vi "set dimmer.vi"(8 "error in":errorcluster, 10 "Set Dim":bool, 11 "Set Max Dim":bool) -> (0 "error out":errorcluster, 3 "Dim Level":T3 scale=0.0..100.0)   [LabVIEW 2013]
uses:
  Controls/Dim level.ctl
  Controls/Power Values.ctl
  <vilib>/addons/Electrical Power/Basic/Measurement/subVIs/basic_Power Value.ctl
  <vilib>/DAQmx/read.llb/DAQmx Read (Analog 1D Wfm NChan NSamp).vi
  <vilib>/addons/Electrical Power/Basic/Measurement/Power (1 Channel).vi
  <vilib>/DAQmx/miscellaneous.llb/DAQmx Fill In Error Info.vi
  <vilib>/addons/Electrical Power/Basic/NI_EP_Basic.lvlib
panel:
  out "Power Values":T1
  out "max dim power":dbl
  out "dim power":dbl
  out "data":waveform(dbl)[](graph)
  # "1) Move dimmer into 100% position and hit \"Set Max Dim\"\n2) Move dimmer to appropriate level, and hit \"Set Dim\""
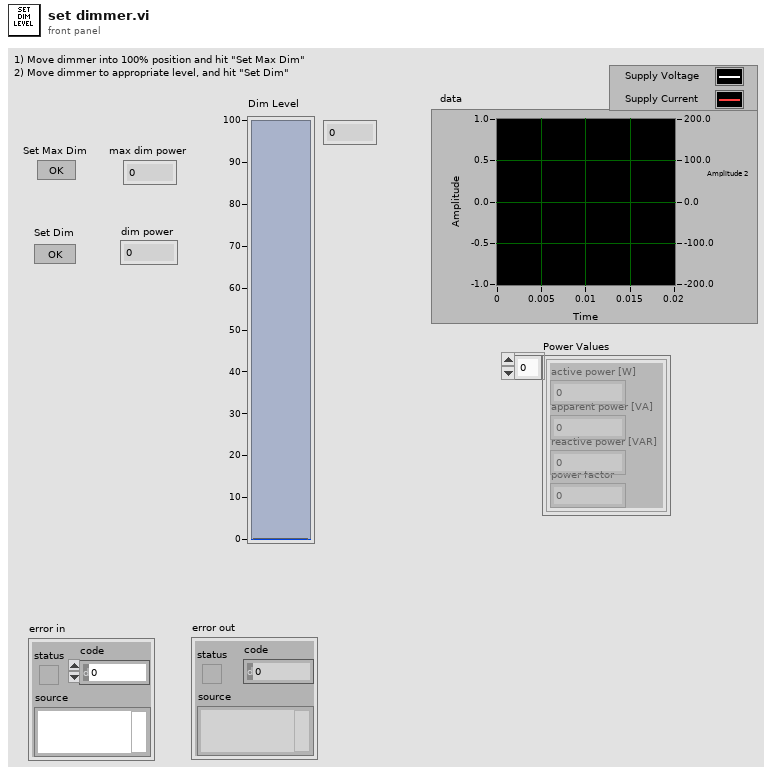
[diagram p1: front panel]
types:
  T1 = typedef "Power Values.ctl" = T2[]
  T2 = typedef "NI_EP_Basic.lvlib/basic_Power Value.ctl" = cluster{"active power [W]":dbl, "apparent power [VA]":dbl, "reactive power [VAR]":dbl, "power factor":dbl}
  T3 = typedef "Dim level.ctl" = dbl
  T4 = enum8{"Enabled", "Disabled", "Disabled and Grayed Out"}
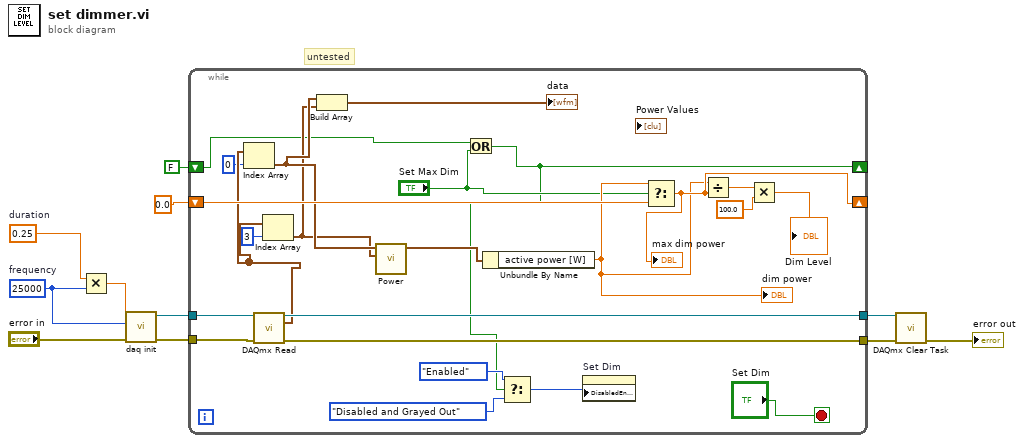
[diagram p0: block diagram]
diagram:
  w3 = 0.25  # duration
  w4 = 25000  # frequency
  # "untested"
  n1 = Multiply(x=w3, y=w4) -> (x*y=w2:dbl)
  n2 = call "daq init.vi"("error in"="error in", "rate"=w4, "number of samples"=w2) -> ("error out"=w8:errorcluster, "task out"=w9:refnum<k21>)  [unwired: 7 in]
  n3 = while {
    tunnel: [w35] -> w11
    tunnel: [w34] -> w10
    tunnel: w9 -> [w33]
    tunnel: w8 -> [w32]
    shift-right: [w29] -> _
    shift-left: 0.0 -> [w31]
    shift-right: [w12] -> _
    shift-left: FALSE -> [w14]
    stop <- "Set Dim" stop-if-true
    n4 = call-poly <vilib>:"DAQmx Read.vi"("task/channels in"=w33, "error in"=w32) -> ("task out"=w34:refnum<k21>, "data"=w24:waveform(dbl)[], "error out"=w35:errorcluster)  [unwired: 11 in]
    n5 = Index Array(array=w24, index=0) -> (element=w21:waveform(dbl))
    n6 = Index Array(array=w24, index=3) -> (element=w20:waveform(dbl))
    n7 = Build Array(w21, w20) -> (→"data":waveform(dbl)[])
    n8 = call-poly <vilib>:"Power.vi"("current waveform"=w20, "voltage waveform"=w21) -> ("power value"=w18:T2)  [unwired: 8 in, 1 out]
    n9 = Or(x=w14, y="Set Max Dim") -> (x .or. y?=w12:bool)
    n10 = Unbundle By Name(w18) -> ("active power [W]"=w25:dbl)
    "dim power" <- w25
    n11 = Select(t=T4."Enabled" ("Disabled"), s=w12, f=T4."Disabled and Grayed Out" ("Disabled")) -> (s? t:f=w15:T4)
    n12 = property on="Set Dim" class="Bool"("DisabledEnum"=w15) -> ()  [unwired: 2 in, 2 out]
    n13 = Select(t=w25, s="Set Max Dim", f=w31) -> (s? t:f=w29:dbl)
    "max dim power" <- w29
    n14 = Divide(x=w25, y=w29) -> (x/y=w28:dbl)
    n15 = Multiply(x=w28, y=100.0) -> (x*y=→"Dim Level":dbl)
  }
  n16 = call <vilib>:"DAQmx Clear Task.vi"("task in"=w10, "error in"=w11) -> ("error out"=→"error out":errorcluster)  [unwired: 13 in]
